vi "MCP23S17_Set.vi"(4 "Data":u32 format="%x", 5 "RF":T1 items=["RF_0", "RF_1", "RF_2", "RF_3"], 6 "Addr":u32, 7 "RFU":T2, 8 "Error_In":errorcluster, 10 "Auto_Sel_Rsrc?":bool=TRUE, 11 "VISA_Rsrc_In":refnum<visa-resource-name>) -> (0 "Error_Out":errorcluster, 3 "VISA_Rsrc_Out":refnum<visa-resource-name>)   [LabVIEW 2018]
uses:
  Types/RFU.ctl
  Types/RF.ctl
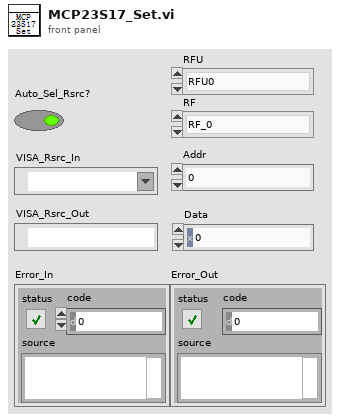
[diagram p1: front panel]
types:
  T1 = typedef "RF.ctl" = u16
  T2 = typedef "RFU.ctl" = enum8{"RFU0", "RFU1", "RFU2", "RFU3", "RFU4"}
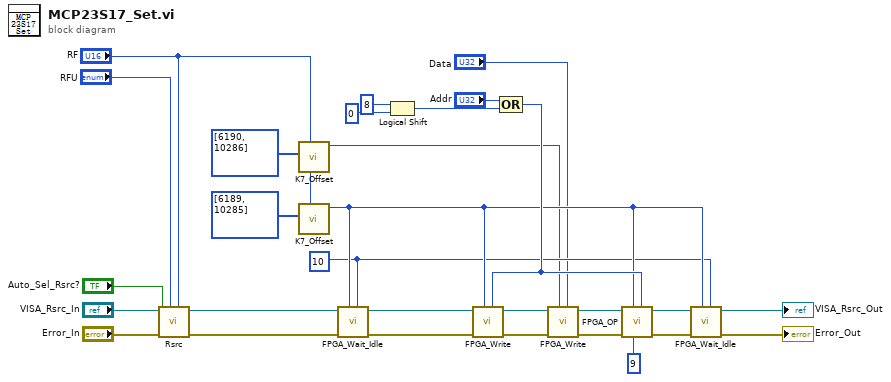
[diagram p0: block diagram]
diagram:
  w11 = u32 10 ("Bit_Offset")
  n1 = call "Rsrc.vi"("RF"="RF", "RFU"="RFU", "Error_In"="Error_In", "Auto_Sel_Rsrc?"="Auto_Sel_Rsrc?", "VISA_Rsrc_In"="VISA_Rsrc_In") -> ("Error_Out"=w28:errorcluster, "VISA_Rsrc_Out"=w24:refnum<visa-resource-name>)  [unwired: 5 in]
  n2 = call "K7_Offset.vi"("RF"="RF", "Offset"=u32[] [6190, 10286]) -> ("Offset"=w7:u32)  [unwired: 9 in]
  n3 = call "K7_Offset.vi"("RF"="RF", "Offset"=u32[] [6189, 10285]) -> ("Offset"=w12:u32)  [unwired: 9 in]
  n4 = call "FPGA_Wait_Idle.vi"("Bit_Offset"=w11, "Offset"=w12, "Error_In"=w28, "VISA_Rsrc_In"=w24) -> ("Error_Out"=w17:errorcluster, "VISA_Rsrc_Out"=w18:refnum<visa-resource-name>)  [unwired: 6 in]
  n5 = Logical Shift(y=i16 8, x=u32 0 ("Bit_Offset")) -> (x << y=w19:u32)
  n6 = Compound Arithmetic op=OR("Addr", w19) -> (w16:u32)
  n7 = call "FPGA_Write.vi"("Value"=w16, "Offset"=w12, "Error_In"=w17, "VISA_Rsrc_In"=w18) -> ("Error_Out"=w8:errorcluster, "VISA_Rsrc_Out"=w9:refnum<visa-resource-name>)  [unwired: 6 in]
  n8 = call "FPGA_Write.vi"("Value"="Data", "Offset"=w7, "Error_In"=w8, "VISA_Rsrc_In"=w9) -> ("Error_Out"=w4:errorcluster, "VISA_Rsrc_Out"=w5:refnum<visa-resource-name>)  [unwired: 6 in]
  n9 = call "FPGA_OP.vi"("Origin_Value"=w16, "OP_Offset"=u32 9, "Offset"=w12, "Error_In"=w4, "VISA_Rsrc_In"=w5) -> ("Error_Out"=w13:errorcluster, "VISA_Rsrc_Out"=w14:refnum<visa-resource-name>)  [unwired: 5 in]
  n10 = call "FPGA_Wait_Idle.vi"("Bit_Offset"=w11, "Offset"=w12, "Error_In"=w13, "VISA_Rsrc_In"=w14) -> ("Error_Out"=→"Error_Out":errorcluster, "VISA_Rsrc_Out"=→"VISA_Rsrc_Out":refnum<visa-resource-name>)  [unwired: 6 in]
